vi "Get Status and Code.vi"(11 "tokens":cluster{"token type":T1, T2}[](array[cluster])) -> (1 "source":string, 2 "code":i32, 3 "status":bool, 4 "substitute":string, 5 "additional":string)   [LabVIEW 2020, in "Multi Error Cluster.lvlib"]
doc: "Given tokens from an error cluster, returnn the core legacy fields."
uses:
  <vilib>/MultiError/TokenizeJSON/Multi Error Cluster.lvlib
  <vilib>/MultiError/TokenizeJSON/JSON Token Values.ctl
  <vilib>/MultiError/Errors Cluster Multiple Errors/JSON Token Descriptor.ctl
  <vilib>/MultiError/TokenizeJSON/JSON Raw Token Values.ctl
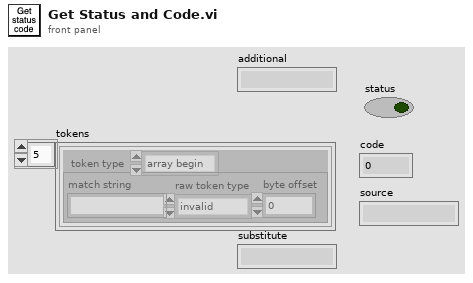
[diagram p1: front panel]
types:
  T1 = typedef "Multi Error Cluster.lvlib/JSON Token Values.ctl" = enum32{"array begin", "array end", "object begin", "object end", "value", "invalid", "name"}
  T2 = typedef "Multi Error Cluster.lvlib/JSON Token Descriptor.ctl" = cluster{"match string":string, "raw token type":T3, "byte offset ":i32}
  T3 = typedef "Multi Error Cluster.lvlib/JSON Raw Token Values.ctl" = enum32{"{", "}", "[", "]", ",", ":", "\"", "number", "string", "true", "false", "null", "invalid"}
  T4 = cluster{"whole match":string, "token index":i32}[]
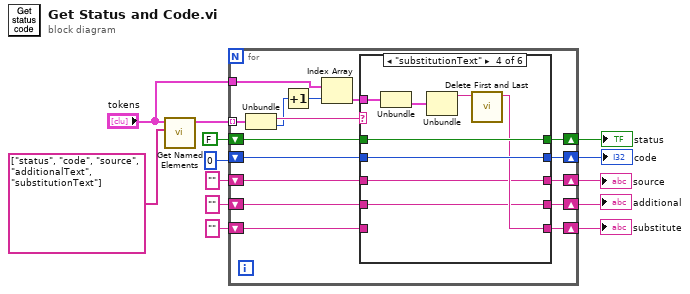
[diagram p0: block diagram]
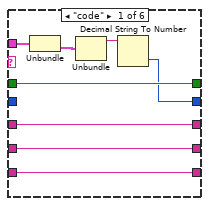
[diagram p2: hidden frame]
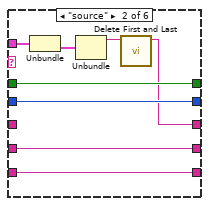
[diagram p3: hidden frame]
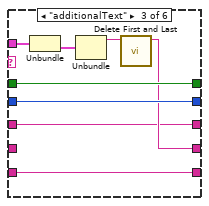
[diagram p4: hidden frame]
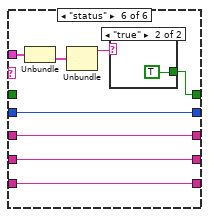
[diagram p6: hidden frame]
diagram:
  n1 = call <vilib>:"Get Named Elements.vi"("names"=string[] ["status", "code", "source", "additionalText", "substitutionText"] ("Names"), "tokens"="tokens") -> ("Found Token Info"=w7:T4)  [unwired: 9 in]
  n2 = for {
    tunnel: w7 -> [w29] mode=indexing
    shift-right: [w26] -> w10
    shift-left: 0 -> [w27]
    shift-right: [w25] -> w9
    shift-left: FALSE -> [w24]
    tunnel: "tokens" -> [w22]
    shift-right: [w19] -> w6
    shift-left: "" ("whole match") -> [w18]
    shift-right: [w14] -> w1
    shift-left: "" ("whole match") -> [w17]
    shift-right: [w15] -> w2
    shift-left: "" ("whole match") -> [w16]
    n3 = Unbundle(w29) -> ("whole match"=w28:string, "token index"=w21:i32)
    n4 = Increment(x=w21) -> (x+1=w23:i32)
    n5 = Index Array(array=w22, index=w23) -> (element=w20:cluster{"token type":T1, T2})
    n6 = case shown="\"substitutionText\"" w28 {
      tunnel: w27 -> [_ w42 w50 w58 w66 w70]
      tunnel: [w33 w42 w50 w58 w66 w70] -> w26
      tunnel: w24 -> [w37 w45 w53 w61 w65 _]
      tunnel: [w37 w45 w53 w61 w65 w71] -> w25
      tunnel: w20 -> [w35 w43 w51 w59 _ w74]
      tunnel: [w32 w40 w47 w54 w64 w69] -> w19
      tunnel: w18 -> [w32 _ w47 w54 w64 w69]
      tunnel: w17 -> [w30 w38 _ w55 w62 w67]
      tunnel: w16 -> [w31 w39 w46 _ w63 w68]
      tunnel: [w31 w39 w46 w56 w63 w68] -> w15
      tunnel: [w30 w38 w48 w55 w62 w67] -> w14
      frame "code" {
        n7 = Unbundle(w35) -> (w36:T2)  [unwired: 1 out]
        n8 = Unbundle(w36) -> ("match string"=w34:string)  [unwired: 2 out]
        n9 = Decimal String To Number(string=w34) -> (number=w33:i32)  [unwired: 2 in, 1 out]
      }
      frame "source" {
        n10 = Unbundle(w43) -> (w44:T2)  [unwired: 1 out]
        n11 = Unbundle(w44) -> ("match string"=w41:string)  [unwired: 2 out]
        n12 = call <vilib>:"Delete First and Last.vi"("string in"=w41) -> ("string subset"=w40:string)  [unwired: 10 in]
      }
      frame "additionalText" {
        n13 = Unbundle(w51) -> (w52:T2)  [unwired: 1 out]
        n14 = Unbundle(w52) -> ("match string"=w49:string)  [unwired: 2 out]
        n15 = call <vilib>:"Delete First and Last.vi"("string in"=w49) -> ("string subset"=w48:string)  [unwired: 10 in]
      }
      frame "substitutionText" {
        n16 = Unbundle(w59) -> (w60:T2)  [unwired: 1 out]
        n17 = Unbundle(w60) -> ("match string"=w57:string)  [unwired: 2 out]
        n18 = call <vilib>:"Delete First and Last.vi"("string in"=w57) -> ("string subset"=w56:string)  [unwired: 10 in]
      }
      frame Default {
      }
      frame "status" {
        n19 = Unbundle(w74) -> (w73:T2)  [unwired: 1 out]
        n20 = Unbundle(w73) -> ("match string"=w72:string)  [unwired: 2 out]
        n21 = case shown="\"true\"" w72 {
          tunnel: [_ TRUE] -> w71
          frame "false", Default {
          }
          frame "true" {
          }
        }
      }
    }
  }
  "code" <- w10
  "status" <- w9
  "source" <- w6
  "additional" <- w1
  "substitute" <- w2
